vi "Time.Get Start of Week.vi"(11 "Time In":timestamp) -> (3 "Start of Week":timestamp)   [LabVIEW 2019]
uses:
  Time.DateTime Adjust Action.ctl
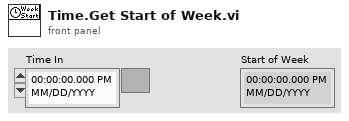
[diagram p1: front panel]
types:
  T1 = typedef "Time.DateTime Adjust Action.ctl" = enum16{"Day Start", "Day End", "Offset Hrs", "UTC to Local", "Local to UTC"}
  T2 = typedef "LVDateTimeRec.ctl" = cluster{"fractional second":dbl, "second":i32, "minute":i32, "hour":i32, "day of month":i32, "month":i32, "year":i32, "day of week":i32, "day of year":i32, "DST":i32}
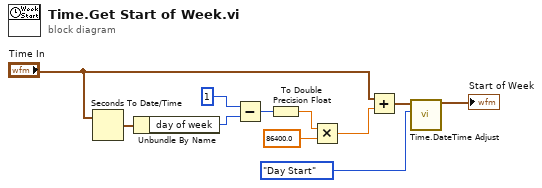
[diagram p0: block diagram]
diagram:
  n1 = Seconds To Date/Time(time stamp (now)="Time In") -> (date time rec=w11:T2)  [unwired: 1 in]
  n2 = Unbundle By Name(w11) -> ("day of week"=w10:i32)
  n3 = Subtract(x=1, y=w10) -> (x-y=w3:i32)
  n4 = To Double Precision Float(number=w3) -> (double precision float=w8:dbl)
  n5 = Multiply(x=w8, y=86400.0) -> (x*y=w6:dbl)
  n6 = Add(x="Time In", y=w6) -> (x+y=w5:timestamp)
  n7 = call "Time.DateTime Adjust.vi"("Action"=Time.DateTime_Adjust_Action."Day Start", "Time Stamp"=w5) -> ("Time Stamp Out"=→"Start of Week":timestamp)  [unwired: 8 in, 1 out]
